vi "Read Data Titles.vi"(8 "error in (no error)":errorcluster, 11 "LakeShore 335 in":refnum<class "LakeShore 335.lvclass">) -> (0 "error out":errorcluster, 2 "Data titles":string[](array[string])=["LS340_T (K)", "LS340_R (Ohm)"], 3 "LakeShore 335 out":refnum<class "LakeShore 335.lvclass">)   [LabVIEW 2014, in "LakeShore 335.lvclass"]
uses:
  LakeShore 335.lvclass
  LakeShore335 Front Panel Data.ctl
  LakeShore335 Heater Ranges.ctl
  Neocera/Neocera Set Point Aproach.ctl
  OO Devices/Device/Read Controls Snapshot.vi
  OO Devices/Device/Read Control Panel Loaded.vi
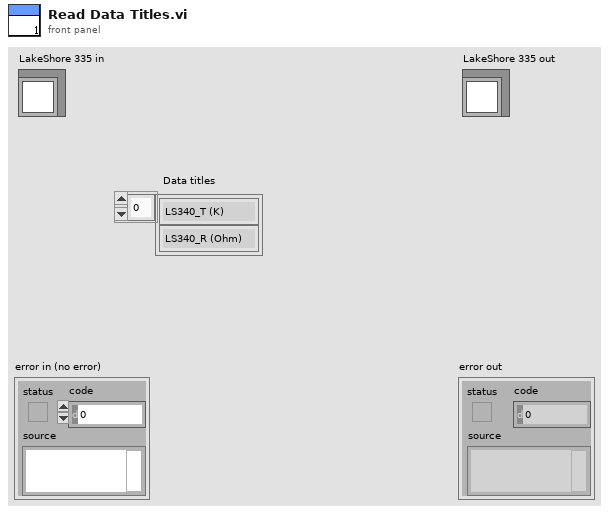
[diagram p1: front panel]
types:
  T1 = typedef "LakeShore335 Front Panel Data.ctl" = cluster{"Heater":bool, "A":bool, "B":bool, " RAW":bool, "Set point":dbl, "Set Heater Range":T2, "Approach":T3, "Ramp rate, K/min":dbl}
  T2 = typedef "LakeShore335 Heater Ranges.ctl" = enum16{"0 (Off)", "1 Low", "2 Medium", "3 High"}
  T3 = typedef "Neocera Set Point Aproach.ctl" = enum16{"Instant", "Ramp"}
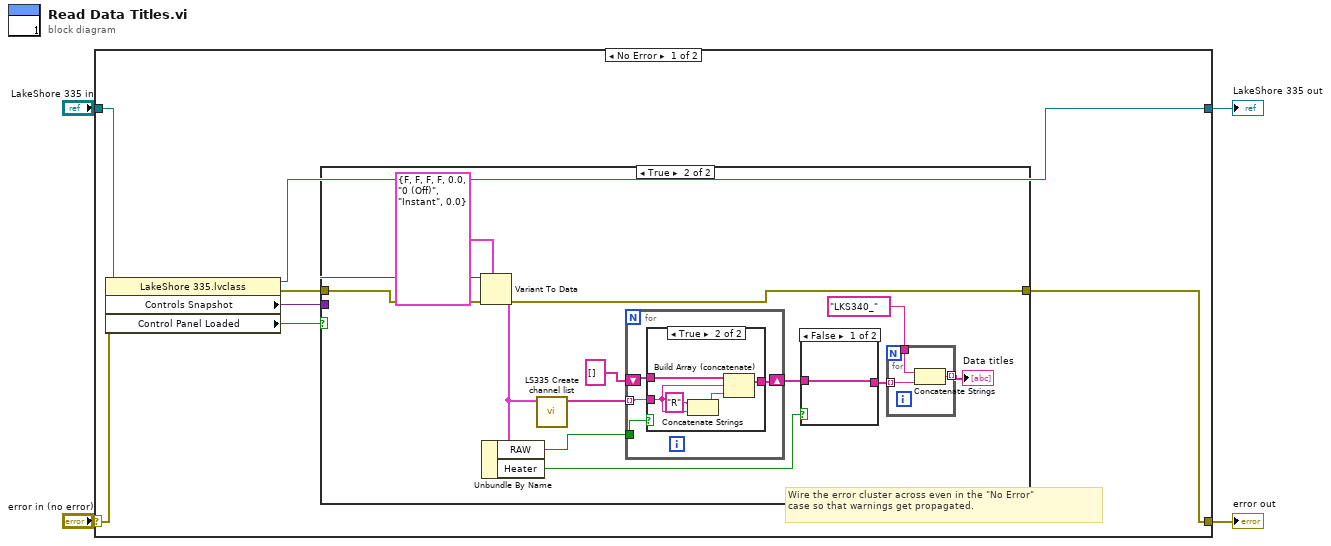
[diagram p0: block diagram]
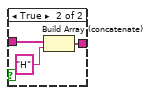
[diagram p3: hidden frame]
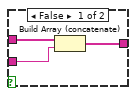
[diagram p4: hidden frame]
diagram:
  n1 = case shown="No Error" "error in (no error)" {
    selector: "error in (no error)" -> [w8 w46]
    tunnel: [w5 w46] -> w3
    tunnel: [w6 w45] -> w1
    tunnel: "LakeShore 335 in" -> [w7 w45]
    frame No Error {
      # "Wire the error cluster across even in the \"No Error\"\ncase so that warnings get propagated."
      n2 = property class="LakeShore 335.lvclass"(reference=w7, error in=w8) -> (reference out=w6:refnum<class "LakeShore 335.lvclass">, error out=w11:errorcluster, "Controls Snapshot"=w10:variant, "Control Panel Loaded"=w9:bool)
      n3 = case shown="True" w9 {
        tunnel: w11 -> [w12 w25]
        tunnel: w10 -> [_ w24]
        tunnel: [w12 w22] -> w5
        frame False {
        }
        frame True {
          n4 = Variant To Data(error in=w25, type=T1 {"Heater"=FALSE, "A"=FALSE, "B"=FALSE, " RAW"=FALSE, "Set point"=0.0, "Set Heater Range"=enum."0 (Off)", "Approach"=enum."Instant", "Ramp rate, K/min"=0.0} ("Data"), Variant=w24) -> (data=w14:T1, error out=w22:errorcluster)
          n5 = Unbundle By Name(w14) -> ("RAW"=w21:bool, "Heater"=w19:bool)
          n6 = call "LS335 Create channel list.vi"("Data"=w14) -> ("Array"=w13:string[])  [unwired: 10 in]
          n7 = for {
            tunnel: w13 -> [w35] mode=indexing
            shift-right: [w36] -> w18
            shift-left: string[] [] -> [w34]
            tunnel: w21 -> [w33]
            n8 = case shown="True" w33 {
              tunnel: [w39 w43] -> w36
              tunnel: w35 -> [w38 w41]
              tunnel: w34 -> [w37 w44]
              frame False {
                n9 = Build Array (concatenate)(w37, w38) -> (w39:string[])
              }
              frame True {
                n10 = Concatenate Strings("R" ("string"), w41) -> (w40:string)
                n11 = Build Array (concatenate)(w44, w41, w40) -> (w43:string[])
              }
            }
          }
          n12 = case shown="False" w19 {
            tunnel: w18 -> [w29 w32]
            tunnel: [w29 w30] -> w17
            frame False {
            }
            frame True {
              n13 = Build Array (concatenate)(w32, "H") -> (w30:string[])
            }
          }
          n14 = for {
            tunnel: "LKS340_" ("string") -> [w28]
            tunnel: w17 -> [w27] mode=indexing
            tunnel: [w26] -> w16 mode=indexing
            n15 = Concatenate Strings(w28, w27) -> (w26:string)
          }
          "Data titles" <- w16
        }
      }
    }
    frame Error {
    }
  }
  "error out" <- w3
  "LakeShore 335 out" <- w1
